vi "Solve2.vi"(8 "Error In":errorcluster, 11 "object in":refnum<class "2022_5.lvclass">) -> (0 "Error Out":errorcluster, 2 "Result":u64, 3 "object out":refnum<class "2022_5.lvclass">)   [LabVIEW 2020, in "2022_5.lvclass"]
uses:
  2022_5.lvclass
  2022_5.lvclass/2022_5.ctl
panel:
  out "TopCrates":string
  out "Move":cluster{"Qty":i32, "From":i32, "To":i32}
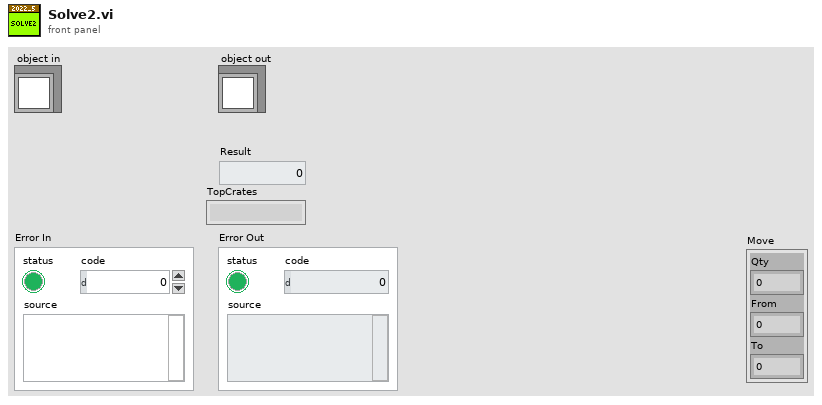
[diagram p1: front panel]
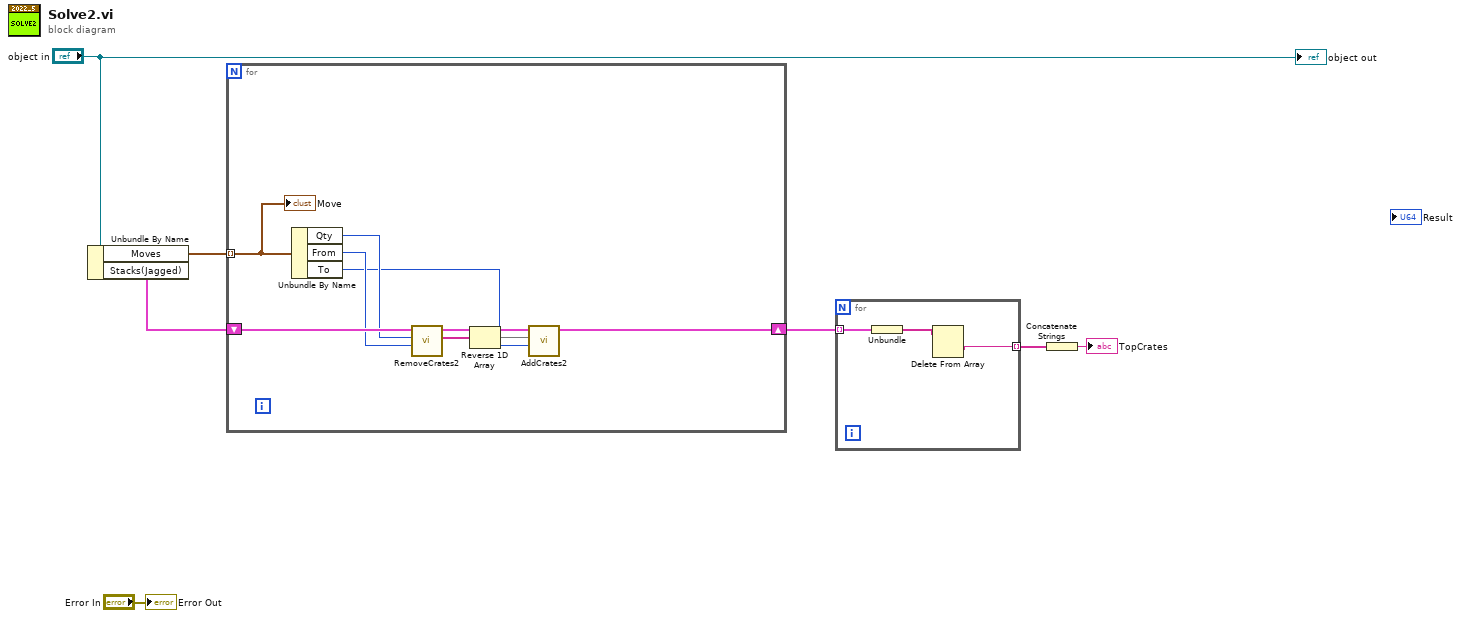
[diagram p0: block diagram]
diagram:
  n1 = Unbundle By Name("object in") -> ("Moves"=w5:cluster{"Qty":i32, "From":i32, "To":i32}[], "Stacks(Jagged)"=w4:cluster{"Crates":string[]}[])
  n2 = for {
    tunnel: w5 -> [w16] mode=indexing
    shift-right: [w11] -> w3
    shift-left: w4 -> [w15]
    n3 = Unbundle By Name(w16) -> ("Qty"=w14:i32, "From"=w13:i32, "To"=w9:i32)
    n4 = call "RemoveCrates2.vi"("From"=w13, "Qty"=w14, "StacksIn"=w15) -> ("CratesRemoved"=w10:string[], "StacksOut"=w12:cluster{"Crates":string[]}[])  [unwired: 7 in]
    n5 = Reverse 1D Array(array=w10) -> (reversed array=w8:string[])
    n6 = call "AddCrates2.vi"("To"=w9, "CratesToAdd"=w8, "StacksIn"=w12) -> ("StacksOut"=w11:cluster{"Crates":string[]}[])  [unwired: 8 in]
    "Move" <- w16
  }
  n7 = for {
    tunnel: w3 -> [w19] mode=indexing
    tunnel: [w17] -> w2 mode=indexing
    n8 = Unbundle(w19) -> ("Crates"=w18:string[])
    n9 = Delete From Array(array=w18) -> (deleted portion=w17:string)  [unwired: 2 in, 1 out]
  }
  n10 = Concatenate Strings(w2) -> (→"TopCrates":string)
  "Error Out" <- "Error In"
  "object out" <- "object in"
